vi "sub_ofdm_packet.vi"(4 "CP length":i32, 6 "FFT size":i32, 8 "message carriers":i32, 9 "pilot symbol":cdb[](array[numeric]), 10 "symbol map":cdb[](array[numeric]), 11 "packet":i8[](array[numeric])) -> (3 "ofdm packet":cdb[](array[numeric]))   [LabVIEW 2014]
uses:
  <vilib>/Analysis/2dsp.llb/Inverse Complex FFT.vi
  <vilib>/addons/Modulation/Digital/General/MT Map Bits to QAM Symbols.vi
  <vilib>/Analysis/NI_AALPro.lvlib
  <vilib>/addons/Modulation/niDMT.lvlib
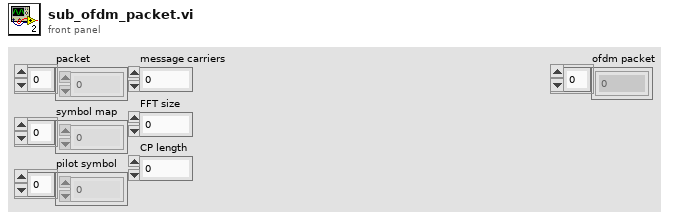
[diagram p1: front panel]
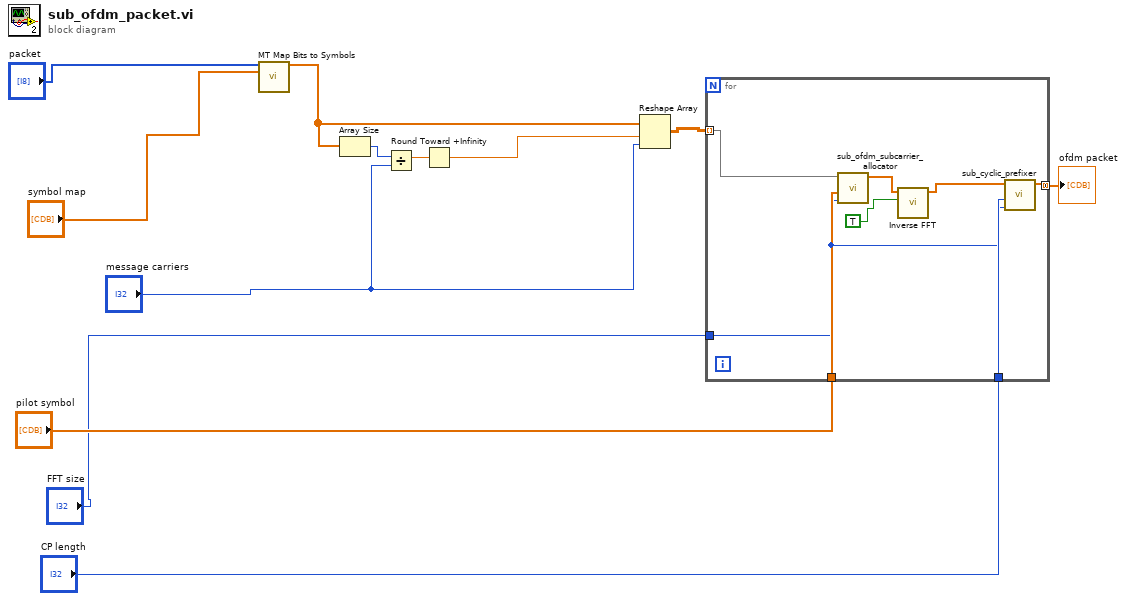
[diagram p0: block diagram]
diagram:
  n1 = call-poly <vilib>:"MT Map Bits to Symbols.vi"("input bit stream"="packet", "symbol map"="symbol map") -> ("symbols"=w5:cdb[])  [unwired: 12 in, 1 out]
  n2 = Array Size(array=w5) -> (size(s)=w4:i32)
  n3 = Divide(x=w4, y="message carriers") -> (x/y=w2:dbl)
  n4 = Round Toward +Infinity(x=w2) -> (ceil(x): smallest int >= x=w1:dbl)
  n5 = Reshape Array(w5, w1, "message carriers") -> (w11:cdb[][])
  n6 = for {
    tunnel: w11 -> [w17] mode=indexing
    tunnel: "pilot symbol" -> [w16]
    tunnel: "FFT size" -> [w14]
    tunnel: "CP length" -> [w15]
    tunnel: [w13] -> w7 mode=concatenating
    n7 = call "sub_ofdm_subcarrier_allocator.vi"("fft size"=w14, "pilot symbol"=w16, "message symbol"=w17) -> ("OFDM symbol"=w18:cdb[])  [unwired: 8 in]
    n8 = call-poly <vilib>:"Inverse FFT.vi"("shift?"=TRUE, "FFT {X}"=w18) -> ("X"=w19:cdb[])  [unwired: 8 in, 1 out]
    n9 = call "sub_cyclic_prefixer.vi"("FFT size"=w14, "CP length"=w15, "time_samples"=w19) -> ("cp ofdm symbol"=w13:cdb[])  [unwired: 8 in]
  }
  "ofdm packet" <- w7
